vi "userauth_keyboard_interactive_response.vi"(8 "error in (no error)":errorcluster, 9 "prompts":T1[](array[typedef]), 10 "instruction":string, 11 "name":string) -> (0 "error out":errorcluster, 2 "responses":string[](array[string]))   [LabVIEW 2017]
doc: "Called when authenticating with libssh2 using <B>libssh2_userauth_keyboard_interactive</B>.\n\n<B>name</B>\n<B>instruction</B> \n<B>prompts</B> challenges provided by the server\n\nReturns the response to the challenges."
uses:
  libssh2/lvssh2_userauth_keyboard_interactive_prompt.ctl
  libssh2/libssh2.lvlib
panel:
  out "Prompt":string
  in  "Password":string
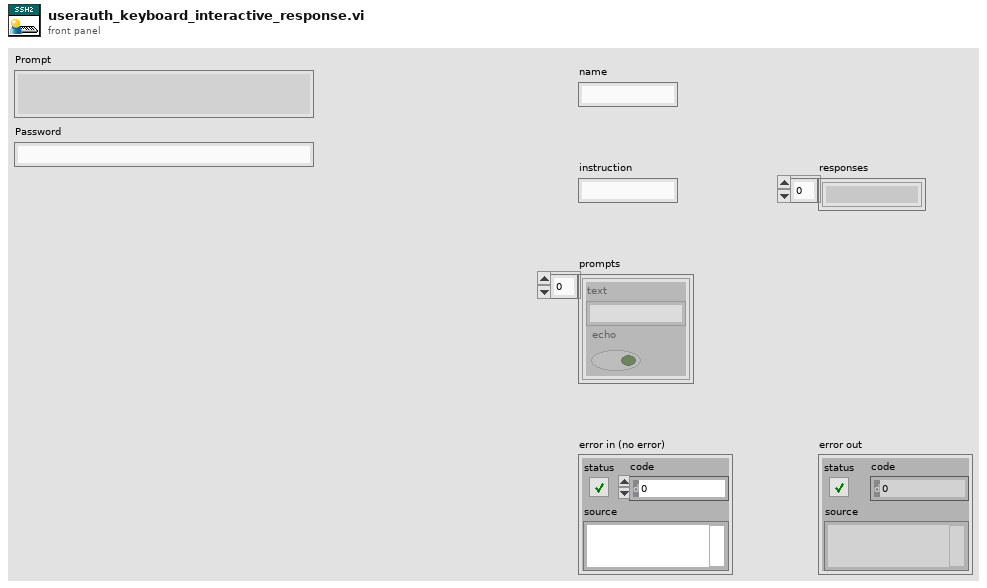
[diagram p1: front panel]
types:
  T1 = typedef "libssh2.lvlib/lvssh2_userauth_keyboard_interactive_prompt.ctl" = cluster{"text":string, "echo":bool}
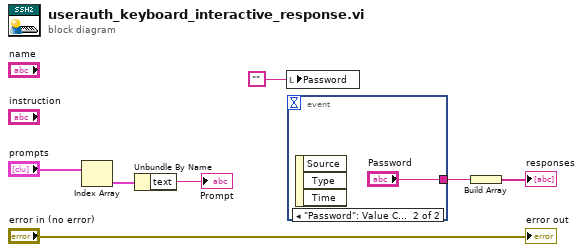
[diagram p0: block diagram]
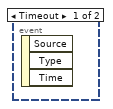
[diagram p2: hidden frame]
diagram:
  n1 = Index Array(array="prompts") -> (element=w3:T1)  [unwired: 1 in]
  n2 = Unbundle By Name(w3) -> ("text"=→"Prompt":string)
  n3 = local write "Password"("") -> ()
  n4 = event shown="[1] \"Password\": Value Change" {
    selector: _ -> [_ _]
    dyn-events: _ -> [_ _]
    timeout: _ -> [_ _]
    tunnel: [_ "Password"] -> w6
    event Timeout {
      n5 = event-data() -> ()  [unwired: 1 in, 3 out]
    }
    event "Password": Value Change {
      n6 = event-data() -> ()  [unwired: 1 in, 3 out]
    }
  }
  n7 = Build Array(w6) -> (→"responses":string[])
  "error out" <- "error in (no error)"
